vi "Destroy User Events.vi"(8 "error in (no error)":errorcluster, 11 "userEvents":T1) -> (0 "error out":errorcluster)   [LabVIEW 2019, in "HLA Custom Device Engine.lvlib" / "User Events.lvlib"]
uses:
  User Events.lvlib
  objectNameNotification_type.ctl
  emea-ni-adg-hla-lv/src/helpers/Dictionaries/_typedefs/lv_dataType_type.ctl
  emea-ni-adg-hla-lv/src/helpers/ObjectManagement/ObjManager.lvlib
  emea-ni-adg-hla-lv/src/helpers/Dictionaries/_typedefs/attribute_type.ctl
  emea-ni-adg-hla-lv/src/helpers/Dictionaries/_typedefs/attribute_map_type.ctl
  emea-ni-adg-hla-lv/src/helpers/Dictionaries/_typedefs/object_type.ctl
  emea-ni-adg-hla-lv/src/helpers/Dictionaries/_typedefs/object_map_type.ctl
  emea-ni-adg-hla-lv/src/helpers/Dictionaries/_typedefs/parameter_type.ctl
  emea-ni-adg-hla-lv/src/helpers/Dictionaries/_typedefs/parameter_map_type.ctl
  emea-ni-adg-hla-lv/src/helpers/Dictionaries/_typedefs/interaction_type.ctl
  emea-ni-adg-hla-lv/src/helpers/Dictionaries/_typedefs/interaction_map_type.ctl
  emea-ni-adg-hla-lv/src/helpers/Dictionaries/_typedefs/instanceHandle_map_type.ctl
  emea-ni-adg-hla-lv/apps/generic/_typedefs/app_data.ctl
  userEvents_type.ctl
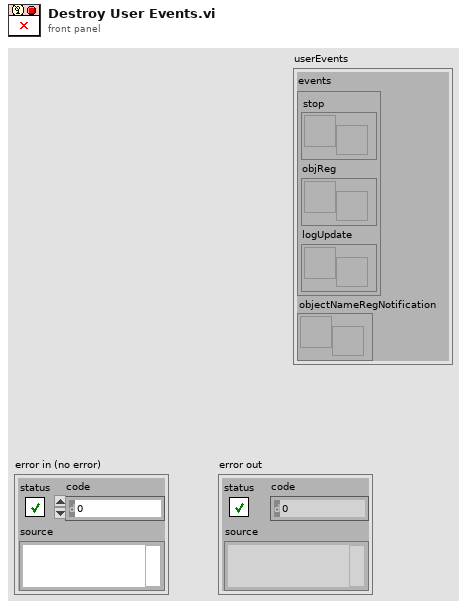
[diagram p1: front panel]
types:
  T1 = typedef "HLA Custom Device Engine.lvlib/User Events.lvlib/userEvents_type.ctl" = cluster{"events":cluster{"stop":refnum<user-event>, "objReg":refnum<user-event>, "logUpdate":refnum<user-event>}, "objectNameRegNotification":refnum<notifier>}
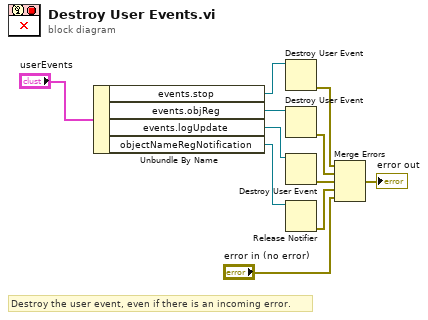
[diagram p0: block diagram]
diagram:
  # "Destroy the user event, even if there is an incoming error."
  n1 = Unbundle By Name("userEvents") -> ("events.stop"=w9:refnum<user-event>, "events.objReg"=w8:refnum<user-event>, "events.logUpdate"=w7:refnum<user-event>, "objectNameRegNotification"=w6:refnum<notifier>)
  n2 = Destroy User Event(user event=w9) -> (error out=w10:errorcluster)  [unwired: 1 in]
  n3 = Destroy User Event(user event=w8) -> (error out=w5:errorcluster)  [unwired: 1 in]
  n4 = Destroy User Event(user event=w7) -> (error out=w4:errorcluster)  [unwired: 1 in]
  n5 = Release Notifier(notifier=w6) -> (error out=w3:errorcluster)  [unwired: 2 in, 2 out]
  n6 = Merge Errors(w10, w5, w4, w3, "error in (no error)") -> (→"error out":errorcluster)
